vi "Doc Builder - Replace Cluster of Keywords.vi"(8 "error in (no error)":errorcluster, 10 "VCluster of KeyVals":variant, 11 "String":string) -> (0 "error out":errorcluster, 3 "String out":string)   [LabVIEW 2011]
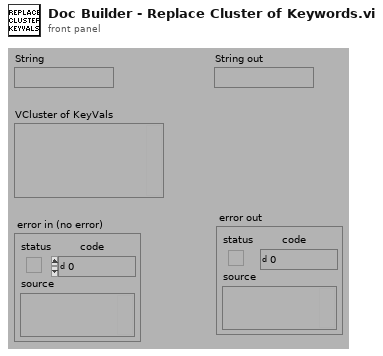
[diagram p1: front panel]
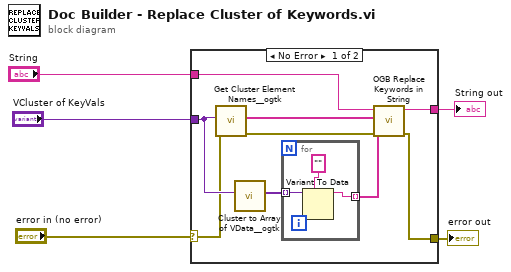
[diagram p0: block diagram]
diagram:
  n1 = case shown="No Error" "error in (no error)" {
    selector: "error in (no error)" -> [w6 w18]
    tunnel: "String" -> [w12 w19]
    tunnel: [w11 w19] -> w2
    tunnel: [w10 w18] -> w3
    tunnel: "VCluster of KeyVals" -> [w9 _]
    frame No Error {
      n2 = call <userlib>:"Get Cluster Element Names__ogtk.vi"("error in (no error)"=w6, "Cluster"=w9) -> ("error out"=w14:errorcluster, "Element Names"=w13:string[])  [unwired: 8 in]
      n3 = call <userlib>:"Cluster to Array of VData__ogtk.vi"("Cluster"=w9) -> ("Array of VData"=w8:variant[])  [unwired: 9 in, 1 out]
      n4 = for {
        tunnel: w8 -> [w17] mode=indexing
        tunnel: [w16] -> w7 mode=indexing
        n5 = Variant To Data(type="" ("String"), Variant=w17) -> (data=w16:string)  [unwired: 1 in, 1 out]
      }
      n6 = call "OGB Replace Keywords in String.vi"("error in (no error)"=w14, "Value"=w7, "Keyword"=w13, "String in"=w12) -> ("error out"=w10:errorcluster, "String out"=w11:string)  [unwired: 6 in]
    }
    frame Error {
    }
  }
  "error out" <- w3
  "String out" <- w2
